vi "ArcadeDrive.vi"(10 "y":dbl, 11 "x":dbl) -> ()   [LabVIEW 2015]
uses:
  <vilib>/Rock Robotics/WPI/RobotDrive/WPI_RobotDriveGetSetRefNum.vi
  <vilib>/Rock Robotics/WPI/RobotDrive/WPI_RobotDriveArcadeDrive_Standard(NoSaturation).vi
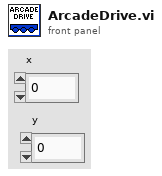
[diagram p1: front panel]
types:
  T1 = typedef "WPI_RobotDriveDevRef.ctl" = cluster{"DevStatus":errorcluster, "Motors[]":T2[], "Square Inputs":bool, "Max Output":dbl}
  T2 = typedef "WPI_MotorControlDeviceRef.ctl" = cluster{"DeviceStatus":errorcluster, "Type":enum16{"PWM", "CAN"}, "PWM":cluster{"Digital Module":T3, "PWM Channel":T4, "DeadBand":T5}, "CAN":cluster{"Device Number":u8, "Control Mode":T6, "Semaphore":T7, "Max Vout":dbl}, "Invert":bool, "TransformRef":T8, "InvTransformRef":T8}
  T3 = typedef "FPGA_TypedefDigitalModule.ctl" = enum16{"Digital Module 1", "Digital Module 2"}
  T4 = typedef "FPGA_DIOPWMChannel.ctl" = enum8{"PWM 1", "PWM 2", "PWM 3", "PWM 4", "PWM 5", "PWM 6", "PWM 7", "PWM 8", "PWM 9", "PWM 10", "Invalid"}
  T5 = typedef "WPI_PWMDeadband.ctl" = cluster{"Name":string, "maxPositivePwm":i32, "minPositivePwm":i32, "centerPwm":i32, "maxNegativePwm":i32, "minNegativePwm":i32, "angularRange":u16}
  T6 = typedef "WPI_CANJaguar_ControlMode.ctl" = enum8{"Percent VBus", "Current", "Speed", "Position", "Voltage"}
  T7 = typedef "Semaphore RefNum" = refnum<k1>
  T8 = typedef "WPI_PWMTransform_ConPane.ctl" = refnum<vi>
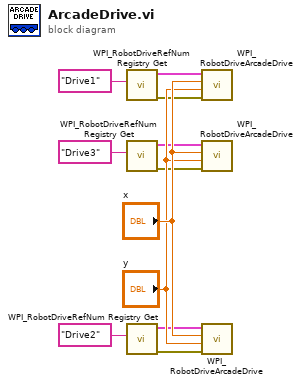
[diagram p0: block diagram]
diagram:
  n1 = call <vilib>:"WPI_RobotDriveRefNum Registry Get.vi"("refnum name"="Drive1") -> ("error out"=w7:errorcluster, "RobotDriveDevRef"=w8:T1)  [unwired: 9 in]
  n2 = call <vilib>:"WPI_RobotDriveRefNum Registry Get.vi"("refnum name"="Drive3") -> ("error out"=w1:errorcluster, "RobotDriveDevRef"=w2:T1)  [unwired: 9 in]
  n3 = call <vilib>:"WPI_RobotDriveRefNum Registry Get.vi"("refnum name"="Drive2") -> ("error out"=w4:errorcluster, "RobotDriveDevRef"=w5:T1)  [unwired: 9 in]
  n4 = call-poly <vilib>:"WPI_RobotDriveArcadeDrive.vi"("error in (no error)"=w7, "Y axis value"="y", "X axis value"="x", "RobotDriveDevRef"=w8) -> ()  [unwired: 5 in, 3 out]
  n5 = call-poly <vilib>:"WPI_RobotDriveArcadeDrive.vi"("error in (no error)"=w1, "Y axis value"="y", "X axis value"="x", "RobotDriveDevRef"=w2) -> ()  [unwired: 5 in, 3 out]
  n6 = call-poly <vilib>:"WPI_RobotDriveArcadeDrive.vi"("error in (no error)"=w4, "Y axis value"="y", "X axis value"="x", "RobotDriveDevRef"=w5) -> ()  [unwired: 5 in, 3 out]
